vi "zadanie 1.vi"() -> ()   [LabVIEW 2018]
panel:
  out "Array":dbl[](array[numeric]) format="%.2f"
  in  "Podzia³":dbl
  in  "podaj N":i32
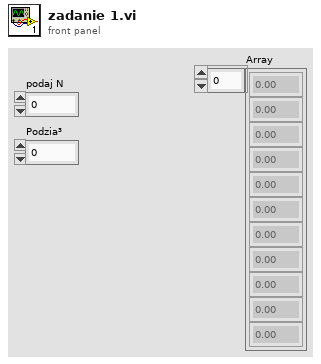
[diagram p1: front panel]
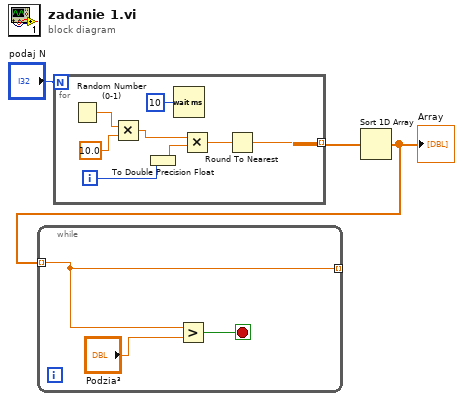
[diagram p0: block diagram]
diagram:
  n1 = for {
    N: "podaj N" -> [_]
    tunnel: [w4] -> w2 mode=indexing
    i -> [w5]
    n2 = Random Number (0-1)() -> (number: 0 to 1=w11:dbl)
    n3 = Multiply(x=w11, y=10.0) -> (x*y=w9:dbl)
    n4 = To Double Precision Float(number=w5) -> (double precision float=w8:dbl)
    n5 = Wait (ms)(milliseconds to wait=u32 10) -> ()  [unwired: 1 out]
    n6 = Multiply(x=w9, y=w8) -> (x*y=w7:dbl)
    n7 = Round To Nearest(number=w7) -> (nearest integer value=w4:dbl)
  }
  n8 = Sort 1D Array(array=w2) -> (sorted array=w1:dbl[])
  "Array" <- w1
  n9 = while {
    tunnel: w1 -> [w14] mode=indexing
    tunnel: [w14] -> _ mode=indexing
    stop <- w12 stop-if-true
    n10 = Greater?(x=w14, y="Podzia³") -> (0:w12:bool)
  }
